vi "Read IPS All.vi"(8 "error in (no error)":errorcluster, 11 "Instrument.VRM in":refnum<class "Instrument.OxfordVRM.lvclass">) -> (0 "error out":errorcluster, 2 "output cluster":T1, 3 "Instrument.VRM out":refnum<class "Instrument.OxfordVRM.lvclass">)   [LabVIEW 2019, in "Instrument.OxfordVRM.lvclass"]
uses:
  Instrument.OxfordVRM.lvclass
  Typedefs/getAll.ctl
  Typedefs/VRM Magnet Axis--Enum.ctl
  Instrument.OxfordVRM.lvclass/Instrument.OxfordVRM.ctl
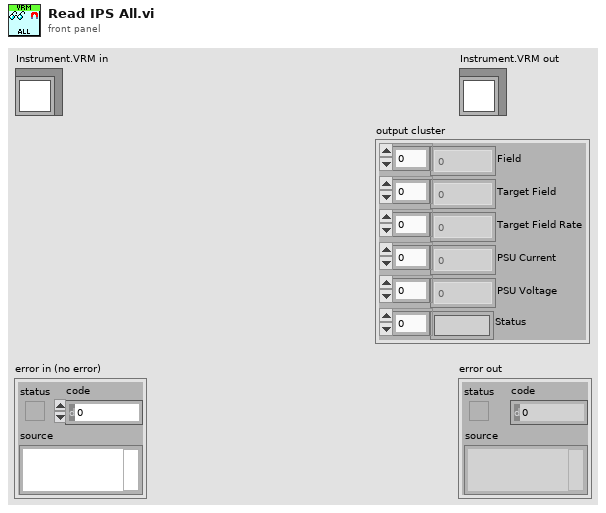
[diagram p1: front panel]
types:
  T1 = typedef "Instrument.OxfordVRM.lvclass/getAll.ctl" = cluster{"Field":dbl[], "Target Field":dbl[], "Target Field Rate":dbl[], "PSU Current":dbl[], "PSU Voltage":dbl[], "Status":string[]}
  T2 = typedef "Instrument.OxfordVRM.lvclass/VRM Magnet Axis--Enum.ctl" = enum16{"X", "Y", "Z", "ALL"}
  T3 = typedef "Instrument.Cryostat.lvclass/Magnet Axis--Enum.ctl" = enum16{"X", "Y", "Z"}
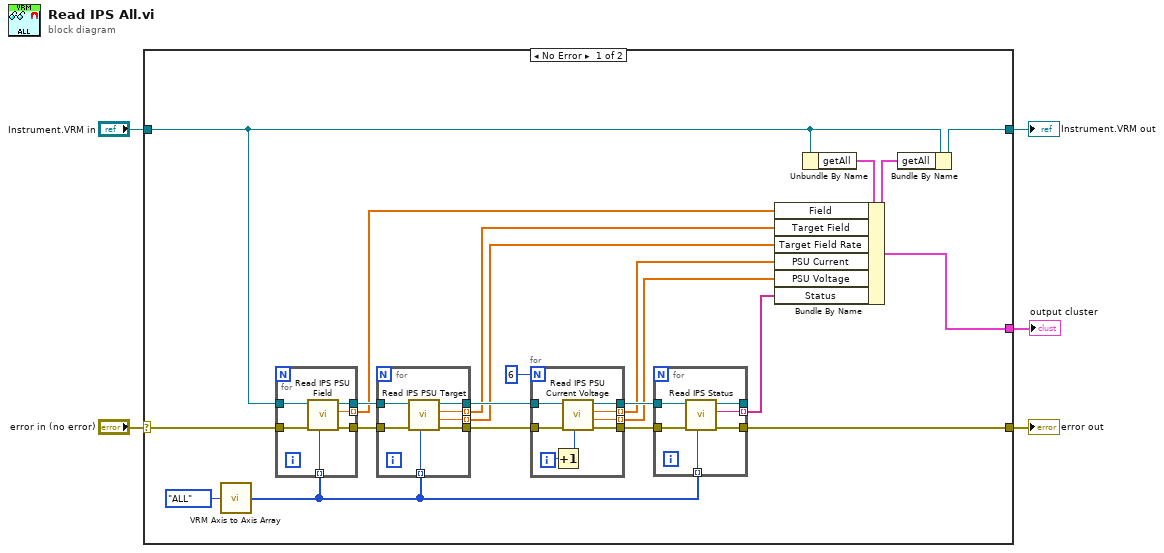
[diagram p0: block diagram]
diagram:
  n1 = case shown="No Error" "error in (no error)" {
    selector: "error in (no error)" -> [w21 w54]
    tunnel: "Instrument.VRM in" -> [w9 w55]
    tunnel: [w10 w55] -> w4
    tunnel: [w12 w54] -> w2
    tunnel: [w6 _] -> w1
    frame No Error {
      n2 = call "VRM Axis to Axis Array.vi"("Axis"=VRM_Magnet_Axis--Enum."ALL") -> ("Axis Array"=w8:T3[])
      n3 = for {
        tunnel: w9 -> [w38]
        tunnel: w21 -> [w37]
        tunnel: [w36] -> w18 mode=indexing
        tunnel: [w35] -> w23
        tunnel: [w34] -> w24
        tunnel: w8 -> [w33] mode=indexing
        n4 = call "Read IPS PSU Field.vi"("Axis"=w33, "error in (no error)"=w37, "Instrument.OxfordVRM in"=w38) -> ("error out"=w35:errorcluster, "Power Supply Field (T)"=w36:dbl, "Instrument.OxfordVRM out"=w34:refnum<class "Instrument.OxfordVRM.lvclass">)  [unwired: 6 in]
      }
      n5 = for {
        tunnel: w24 -> [w45]
        tunnel: w23 -> [w44]
        tunnel: [w43] -> w17 mode=indexing
        tunnel: [w42] -> w16 mode=indexing
        tunnel: [w41] -> w25
        tunnel: [w40] -> w22
        tunnel: w8 -> [w39] mode=indexing
        n6 = call "Read IPS PSU Target.vi"("Axis"=w39, "error in (no error)"=w44, "Instrument.OxfordVRM in"=w45) -> ("error out"=w40:errorcluster, "Target Field Rate (T/min)"=w42:dbl, "Target Field (T)"=w43:dbl, "Instrument.OxfordVRM out"=w41:refnum<class "Instrument.OxfordVRM.lvclass">)  [unwired: 5 in]
      }
      n7 = for {
        N: 6 -> [_]
        tunnel: w25 -> [w53]
        tunnel: w22 -> [w52]
        tunnel: [w50] -> w15 mode=indexing
        tunnel: [w49] -> w14 mode=indexing
        tunnel: [w48] -> w20
        tunnel: [w47] -> w19
        i -> [w51]
        n8 = Increment(x=w51) -> (x+1=w46:i32)
        n9 = call "Read IPS PSU Current Voltage.vi"("PSU #"=w46, "error in (no error)"=w52, "Instrument.OxfordVRM in"=w53) -> ("error out"=w47:errorcluster, "Voltage (V)"=w49:dbl, "Current (A)"=w50:dbl, "Instrument.OxfordVRM out"=w48:refnum<class "Instrument.OxfordVRM.lvclass">)  [unwired: 5 in]
      }
      n10 = for {
        tunnel: w20 -> [w32]
        tunnel: w19 -> [w31]
        tunnel: [w30] -> w13 mode=indexing
        tunnel: [w29] -> _
        tunnel: [w28] -> w12
        tunnel: w8 -> [w27] mode=indexing
        n11 = call "Read IPS Status.vi"("Axis"=w27, "error in (no error)"=w31, "Instrument.OxfordVRM in"=w32) -> ("error out"=w28:errorcluster, "Status"=w30:string, "Instrument.OxfordVRM out"=w29:refnum<class "Instrument.OxfordVRM.lvclass">)  [unwired: 6 in]
      }
      n12 = Unbundle By Name(w9) -> ("getAll"=w26:T1)
      n13 = Bundle By Name(cluster=w26, "Field"=w18, "Target Field"=w17, "Target Field Rate"=w16, "PSU Current"=w15, "PSU Voltage"=w14, "Status"=w13) -> (w6:T1)
      n14 = Bundle By Name(cluster=w9, "getAll"=w6) -> (w10:refnum<class "Instrument.OxfordVRM.lvclass">)
    }
    frame Error {
    }
  }
  "error out" <- w2
  "Instrument.VRM out" <- w4
  "output cluster" <- w1
